vi "getNonOverlapIdx.vi"(0 "Input Idx Array":i32[](array[numeric]), 2 "Overlap Idx Array":i32[](array[numeric])) -> (7 "Non-Overlap Idx Array":i32[](array[numeric]))   [LabVIEW 2016]
doc: "Get the non overlap index array from the input index array."
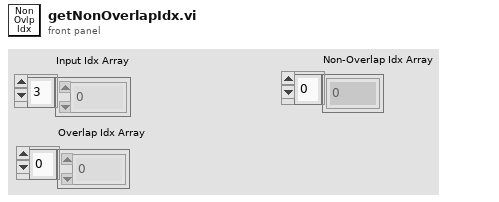
[diagram p1: front panel]
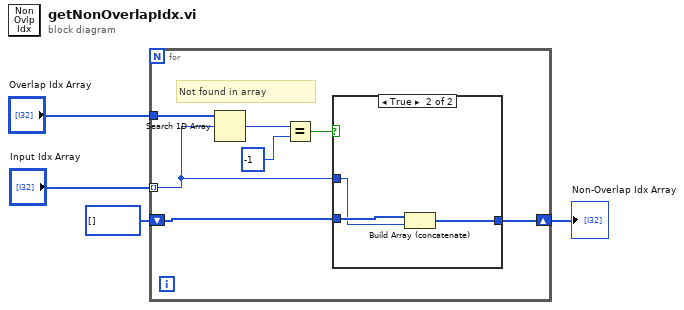
[diagram p0: block diagram]
diagram:
  n1 = for {
    tunnel: "Overlap Idx Array" -> [w11]
    tunnel: "Input Idx Array" -> [w7] mode=indexing
    shift-right: [w5] -> w2
    shift-left: i32[] [] -> [w6]
    # "Not found in array"
    n2 = Search 1D Array(1D array=w11, element=w7) -> (index of element=w10:i32)  [unwired: 1 in]
    n3 = Equal?(x=w10, y=-1) -> (x = y?=w8:bool)
    n4 = case shown="True" w8 {
      tunnel: w7 -> [_ w13]
      tunnel: w6 -> [w12 w15]
      tunnel: [w12 w14] -> w5
      frame False {
      }
      frame True {
        n5 = Build Array (concatenate)(w15, w13) -> (w14:i32[])
      }
    }
  }
  "Non-Overlap Idx Array" <- w2
